vi "try motor.vi"() -> ()   [LabVIEW 2009]
uses:
  User Interface/buttons pressed.ctl
  <vilib>/NXT/Dual Mode Library/Display/drawText.vi
  <vilib>/NXT/Dual Mode Library/prims/inRangeAndCoerce/inRangeAndCoerce_int.vi
  <vilib>/NXT/Dual Mode Library/Sensors/Read_Battery.vi
  <vilib>/NXT/Subs/MotorOutput.ctl
  <vilib>/NXT/Dual Mode Library/Motors/MotorOn.vi
  <vilib>/NXT/HiTechnic/TETRIX Move DC Motors (single).vi
panel:
  out "Power":string
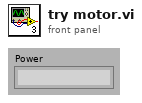
[diagram p1: front panel]
types:
  T1 = typedef "buttons pressed.ctl" = u8
  T2 = typedef "LVHSConnector.ctl" = cluster{"error":errorcluster, "address":string, "NXT #":i32, "Show Error":bool, "Connection":u16}
  T3 = typedef "MotorOutput.ctl" = u8
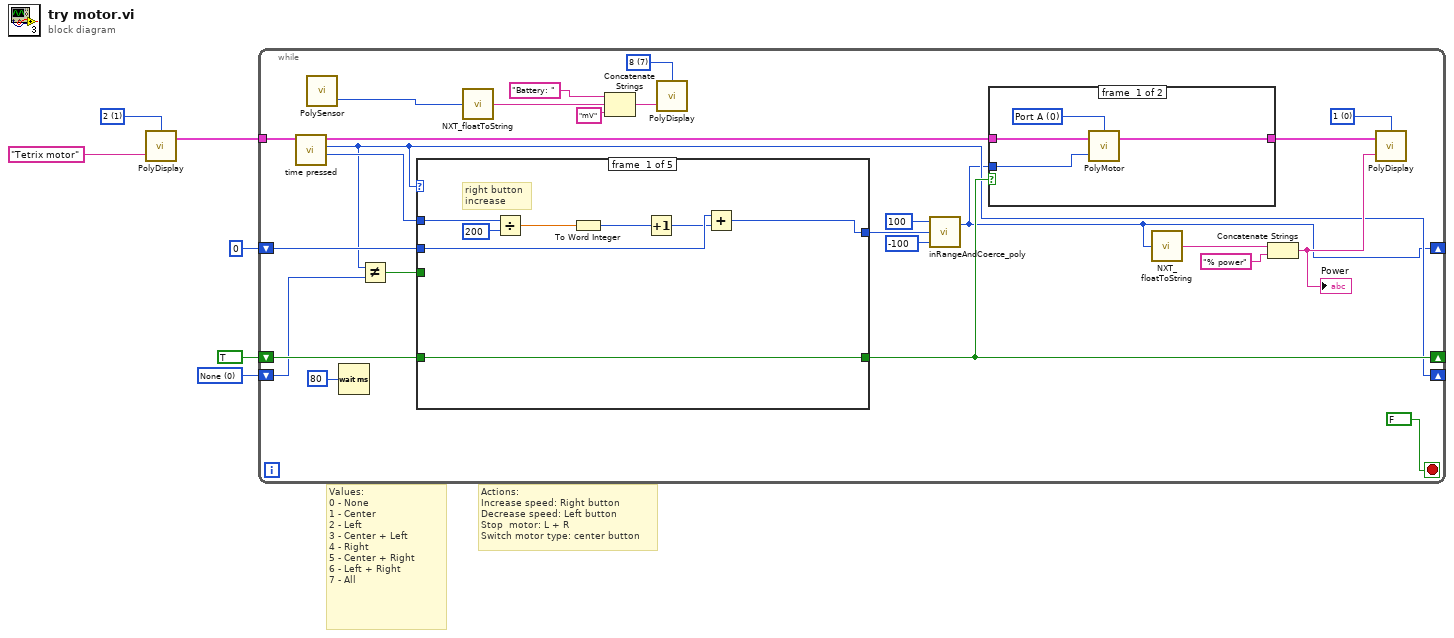
[diagram p0: block diagram]
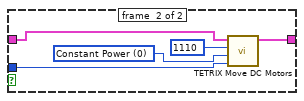
[diagram p2: hidden frame]
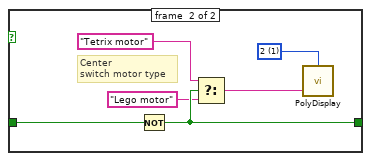
[diagram p4: hidden frame]
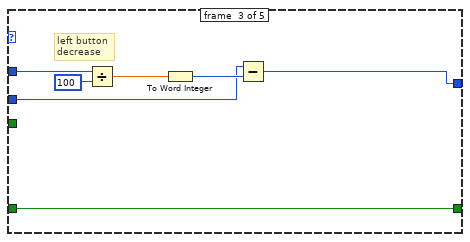
[diagram p5: hidden frame]
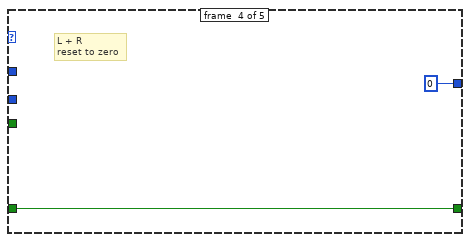
[diagram p6: hidden frame]
diagram:
  w3 = i16 1 items=["1", "2", "3", "4", "5", "6", "7", "8"] ("Line")
  w4 = T1 0 items=["None", "Center", "Left", "C+L", "Right", "C+R", "C+L", "All"] ("Buttons pressed")
  # "Actions:\nIncrease speed: Right button\nDecrease speed: Left button\nStop  motor: L + R\nSwitch motor type: center button"
  # "Values:\n0 - None\n1 - Center\n2 - Left\n3 - Center + Left\n4 - Right\n5 - Center + Right\n6 - Left + Right\n7 - All"
  n1 = call-poly <vilib>:"PolyDisplay.vi"("Text"="Tetrix motor", "Line"=w3) -> ("NXT"=w2:T2)  [unwired: 2 in]
  n2 = while {
    shift-right: [w16] -> _
    shift-left: i16 0 ("Power/Speed") -> [w32]
    shift-right: [w23] -> _
    shift-left: TRUE -> [w24]
    shift-right: [w19] -> _
    shift-left: w4 -> [w21]
    tunnel: w2 -> [w13]
    stop <- FALSE stop-if-true
    w8 = i16 7 items=["1", "2", "3", "4", "5", "6", "7", "8"] ("Line")
    w28 = i16 0 items=["1", "2", "3", "4", "5", "6", "7", "8"] ("Line")
    n3 = call "time pressed.vi"("NXT"=w13) -> ("time pressed (ms)"=w22:u32, "Buttons pressed"=w19:T1, "NXT 2"=w31:T2)  [unwired: 8 in]
    n4 = call-poly <vilib>:"PolySensor.vi"() -> ("millivolts"=w7:i16)  [unwired: 3 in, 1 out]
    n5 = Wait (ms)(milliseconds to wait=u32 80) -> ()  [unwired: 1 out]
    n6 = Not Equal?(x=w19, y=w21) -> (x != y?=w20:bool)
    n7 = case shown="1" w19 {
      tunnel: [w44 w51 w62 i16 0 ("Power/Speed") w71] -> w17
      tunnel: w32 -> [w45 w51 w63 _ w71]
      tunnel: w22 -> [w49 _ w67 _ _]
      tunnel: [w43 w52 w61 w68 w70] -> w23
      tunnel: w24 -> [w43 w53 w61 w68 w70]
      tunnel: w20 -> [_ w50 _ _ _]
      frame #0 {
        # "right button\nincrease"
        n8 = Divide(x=w49, y=u32 200) -> (x/y=w47:dbl)
        n9 = To Word Integer(number=w47) -> (16bit integer=w46:i16)
        n10 = Increment(x=w46) -> (x+1=w42:i16)
        n11 = Add(x=w45, y=w42) -> (x+y=w44:i32)
      }
      frame #1 {
        n12 = case shown="True" w50 {
          tunnel: w53 -> [w54 w60]
          tunnel: [w54 w58] -> w52
          frame #0 {
          }
          frame #1 {
            w59 = i16 1 items=["1", "2", "3", "4", "5", "6", "7", "8"] ("Line")
            # "Center\nswitch motor type"
            n13 = Not(x=w60) -> (.not. x?=w58:bool)
            n14 = Select(t="Tetrix motor", s=w58, f="Lego motor") -> (s? t:f=w55:string)
            n15 = call-poly <vilib>:"PolyDisplay.vi"("Text"=w55, "Line"=w59) -> ()  [unwired: 2 in, 1 out]
          }
        }
      }
      frame #2 {
        # "left button\ndecrease"
        n16 = Divide(x=w67, y=u32 100) -> (x/y=w65:dbl)
        n17 = To Word Integer(number=w65) -> (16bit integer=w64:i16)
        n18 = Subtract(x=w63, y=w64) -> (x-y=w62:i32)
      }
      frame #3 {
        # "L + R\nreset to zero"
      }
      frame #4 {
      }
    }
    n19 = call <vilib>:"NXT_floatToString.vi"("number"=w7) -> ("string"=w10:string)
    n20 = Concatenate Strings("Battery: ", w10, "mV") -> (w9:string)
    n21 = call-poly <vilib>:"PolyDisplay.vi"("Text"=w9, "Line"=w8) -> ()  [unwired: 2 in, 1 out]
    n22 = call-poly <vilib>:"inRangeAndCoerce_poly.vi"("lower limit"=-100, "x"=w17, "upper limit"=100) -> ("coerced(x)"=w16:i32)  [unwired: 1 out]
    n23 = case shown="True" w23 {
      tunnel: w31 -> [w36 w39]
      tunnel: [w35 w38] -> w29
      tunnel: w16 -> [w33 w37]
      frame #0 {
        w34 = T3 0 items=["Port A", "Port B", "Port C", "All Ports"] ("Output Port (All Ports)")
        n24 = call-poly <vilib>:"PolyMotor.vi"("Power (75)"=w33, "NXT"=w36, "Output Port (All Ports)"=w34) -> ("NXT"=w35:T2)  [unwired: 1 in]
      }
      frame #1 {
        w40 = u8 0 items=["Constant Power", "Constant Speed"] ("Control Mode (Constant Power)")
        n25 = call-poly <vilib>:"TETRIX Move DC Motors.vi"("Power/Speed"=w37, "Control Mode (Constant Power)"=w40, "DC Motor"=u32 1110, "NXT"=w39) -> ("NXT"=w38:T2)  [unwired: 7 in]
      }
    }
    n26 = call <vilib>:"NXT_floatToString.vi"("number"=w16) -> ("string"=w27:string)
    n27 = Concatenate Strings(w27, "% power" ("string")) -> (w26:string)
    "Power" <- w26
    n28 = call-poly <vilib>:"PolyDisplay.vi"("Text"=w26, "NXT"=w29, "Line"=w28) -> ()  [unwired: 1 in, 1 out]
  }
